vi "ODH_LEGO_Programatically_Open_Consumer.vi"(8 "Error In":errorcluster, 11 "vi path":path=path "D:/Licenta/LEGO_Comfort_Close_Sensor_Activation.vi") -> (0 "Error Out":errorcluster={"status"=TRUE, "code"=1000, "source"="Invoke Node in ODH_LEGO_Programatically_Open_Consumer.vi->ODH_LEGO_Programatically_Open_Consumer.vi.ProxyCaller\n<APPEND>\nMethod Name: <b>Run VI</b>\n\nVI Path: <b>C:\\ODH_Automated_Test_Setup\\Lego\\ODH_LEGO_Consumer.vi</b>"})   [LabVIEW 2016]
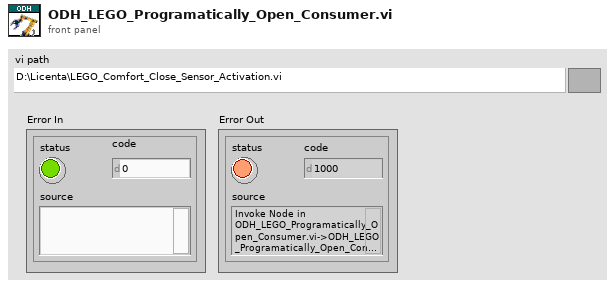
[diagram p1: front panel]
types:
  T1 = enum32{"Bad", "Idle", "Run top level", "Running"}
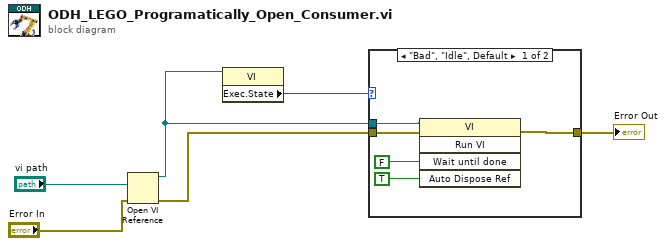
[diagram p0: block diagram]
diagram:
  n1 = Open VI Reference(vi path="vi path", error in (no error)="Error In") -> (vi reference=w3:refnum<vi>, error out=w5:errorcluster)  [unwired: 4 in]
  n2 = property class="VI"(reference=w3) -> ("Exec.State"=w2:T1)  [unwired: 1 in, 2 out]
  n3 = case shown="\"Bad\", \"Idle\", Default" w2 {
    tunnel: w5 -> [w8 w12]
    tunnel: w3 -> [w9 _]
    tunnel: [w7 w12] -> w1
    frame "Bad", "Idle", Default {
      n4 = invoke class="VI" method="Run VI"(reference=w9, error in=w8, "Wait until done"=FALSE ("Wait Until Done"), "Auto Dispose Ref"=TRUE ("Auto Dispose Reference")) -> (error out=w7:errorcluster)  [unwired: 1 in, 4 out]
    }
    frame "Run top level", "Running" {
    }
  }
  "Error Out" <- w1
